vi "Dashboard Main.vi"() -> ()   [LabVIEW 2013]
uses:
  <vilib>/event_ctls.llb/eventvkey.ctl
  <vilib>/Utility/config.llb/Read Key (String).vi
  <vilib>/Utility/config.llb/Read Key (I32).vi
  <vilib>/Utility/config.llb/Write Key (String).vi
  <vilib>/Utility/config.llb/Write Key (I32).vi
  <vilib>/Utility/config.llb/NI_LVConfig.lvlib
panel:
  in  "Switches":bool
  out "Battery Value":dbl(slide) scale=0.0..14.0 scale format="%#_2e"
  out "Battery":sgl(graph)
  in  "Camera Settings":T1={"Frate Rate"=30, "Compression"=30, "Size"=1} {"Frate Rate" scale=1.0..30.0; "Size" items=["640x480", "320x240", "160x120"]}
  out "Mode":T2(ring)=enum."Auto Disabled"
  out "Camera IP":string
  out "JS1 Z":dbl(slide) scale=-1.0..1.0 scale format="%#_2e"
  out "JS2 Z":dbl(slide) scale=-1.0..1.0 scale format="%#_2e"
  out "Joystick 1":cluster{"X":dbl, "Y":dbl}[](graph)
  out "Joystick 2":cluster{"X":dbl, "Y":dbl}[](graph)
  out "JS Buttons 1":T3
  out "JS Buttons 2":T3
  out "MotorSlide4":dbl(slide) scale=-1.0..1.0 scale format="%#_2e"
  out "MotorSlide3":dbl(slide) scale=-1.0..1.0 scale format="%#_2e"
  out "MotorSlide2":dbl(slide) scale=-1.0..1.0 scale format="%#_2e"
  in  "MotorName3":string="Front Left"
  in  "MotorName4":string="Front Right"
  in  "MotorName1":string="Rear Left"
  in  "MotorName2":string="Rear Right"
  out "MotorChart4":dbl(graph)
  out "MotorChart3":dbl(graph)
  out "MotorChart2":dbl(graph)
  out "MotorSlide1":dbl(slide) scale=-1.0..1.0 scale format="%#_2e"
  out "MotorChart1":dbl(graph)
  out "Robot IP":string
  in  "Dashboard Tab":enum32{"Camera Image", "Test", "Checklist"}(tab)
  out "Right Claw 2":bool
  out "Left Claw":bool
  out "Right MAX":bool
  out "Left MAX":bool
  out "Shooter MIN":bool
  in  "Slider":dbl(slide) scale=0.0..100.0 scale format="%#_3g"
  in  "On/Off":bool caption="Solenoid"
  in  "Test Name":u16(ring) items=["Select the test to run...", "Example Test", "-------------------------------", "List of tests is built in robot code.", "Replace with your own automated tests."]
  in  "Test Tree":string(tree)
  in  "Motor":cluster{"Value":dbl, "Enable":bool} {"Value" scale=-1.0..1.0 scale format="%#_3g"}
  out "Progress":T4 {"Test Progress" scale=0.0..100.0}
  in  "Rev/Fwd":cluster{"Forward":bool, "Reverse":bool}
  in  "Ring":u16(ring) items=["Auto", "Fixed indoor", "Fixed outdoor 1", "Fixed outdoor 2", "Fixed fluorescent 1", "Fixed fluorescent 2", "Hold current"]
  in  "Listbox":i32(listbox)
  in  "Viewer":enum32{"Operation", "Variables"}(tab)
  out "Image Error Message":string="Timeout in Camera Communications"
  out "fps":dbl format="%#.1g"
  out "Mbps 2":bool
  in  "DB Camera Config":bool
  in  "Enable":bool
  out "Mbps":dbl format="%#.1g"
  out "Camera Image":T5(plugin-control)
  out "Tree":string(tree)
  # "Drive & Motors"
  # "Robot IP:"
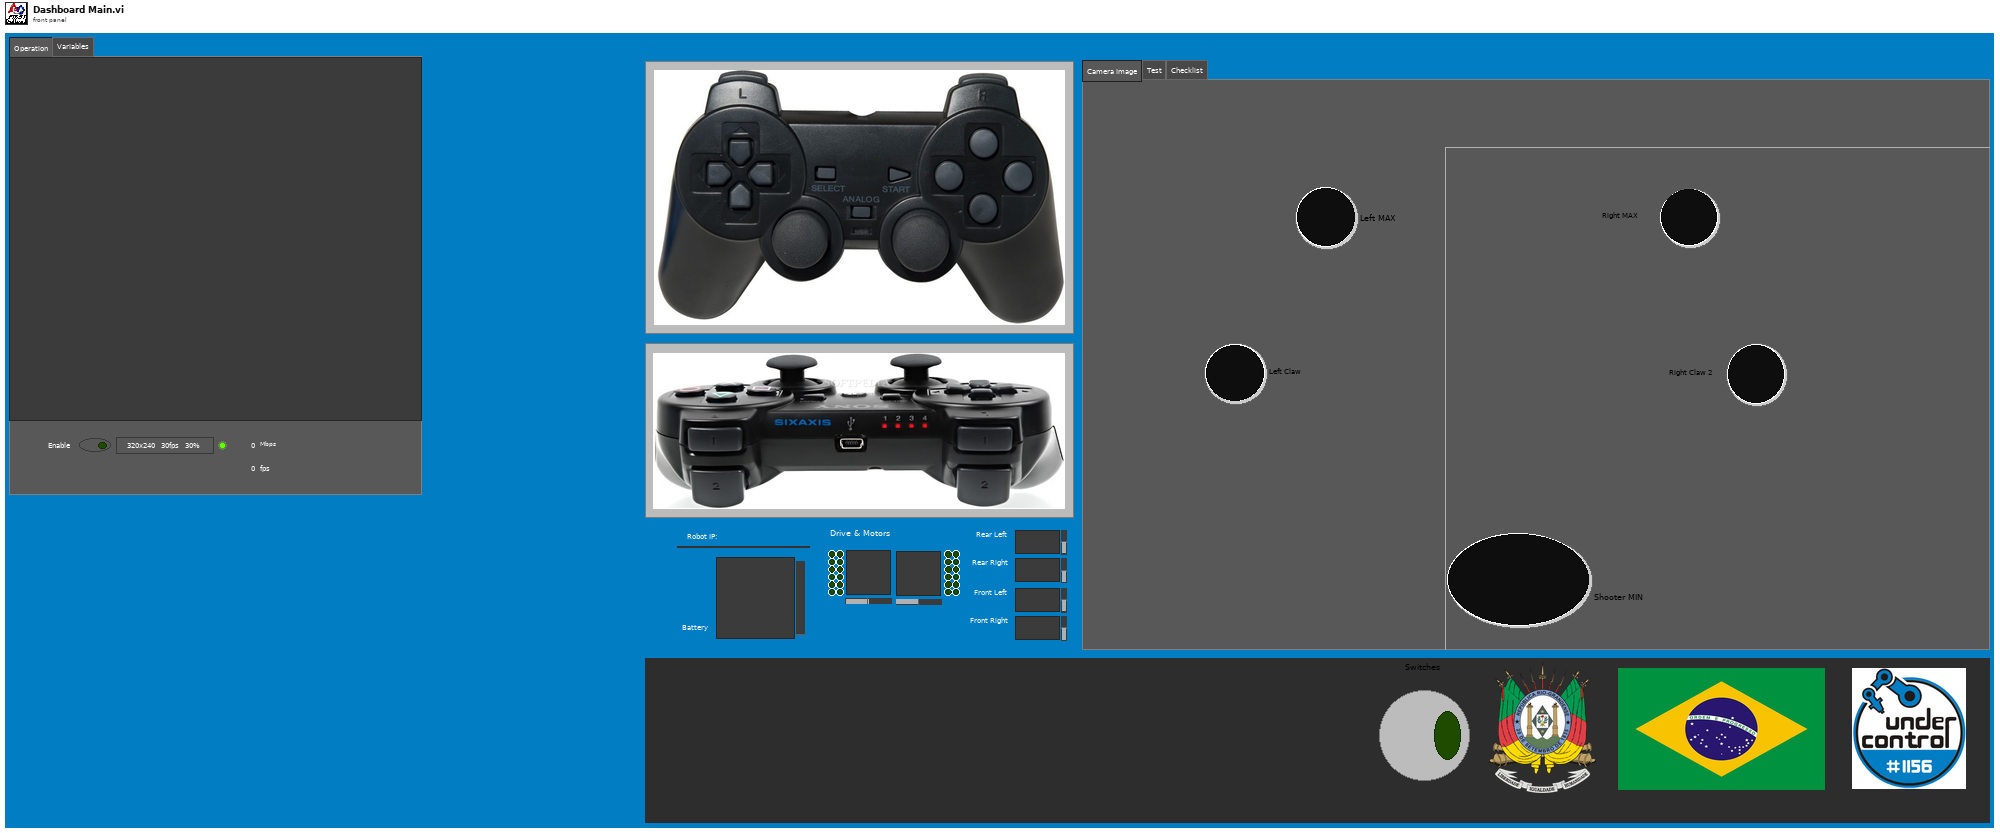
[diagram p1: front panel]
types:
  T1 = cluster{"Frate Rate":i32, "Compression":i32, "Size":u16}
  T2 = enum8{"Tele-Op Disabled", "Tele-Op Enabled", "Auto Disabled", "Auto Enabled", "Test Disabled", "Test Enabled", ""}
  T3 = cluster{bool, bool, bool, bool, bool, bool, bool, bool, bool, bool, bool, bool}
  T4 = cluster{"Test Progress":u8, "Test Progress Text":string}
  T5 = typedef "IMAQ Image.ctl" = refnum<image>
  T6 = typedef "Image Type" = u32
  T7 = typedef "LVRectTypeDef.ctl" = cluster{"Left":i16, "Top":i16, "Right":i16, "Bottom":i16}
  T8 = cluster{"Competition mode":bool, "Robot Link":bool, "Autonomous":bool, "Enabled":bool, "E-Stop":bool, "Simulated":bool, "TestMode":bool, "Docked Window":bool}
  T9 = cluster{"Boolean Array[0]":bool, "Boolean Array[1]":bool, "Boolean Array[2]":bool, "Boolean Array[3]":bool, "Boolean Array[4]":bool, "Boolean Array[5]":bool, "Boolean Array[6]":bool, "Boolean Array[7]":bool, "Boolean Array[8]":bool, "Boolean Array[9]":bool, "Boolean Array[10]":bool, "Boolean Array[11]":bool}
  T10 = typedef "NI_LVConfig.lvlib/Config Data RefNum.ctl" = refnum<k1>
  T11 = typedef "eventvkey.ctl" = enum16{"ASCII", "Enter", "Return", "Shift", "Ctrl", "Alt", "Cmd", "Opt", "Caps", "NumLock", "Clear", "Break", "Up", "Down", "Left", "Right", "Insert", "Delete", "Home", "End", "PageUp", "PageDown", "Escape", "Help", "Pause", "ScrollLock", "F1", "F2", "F3", "F4", "F5", "F6", "F7", "F8", "F9", "F10", "F11", "F12", "F13", "F14", "F15", "F16", "F17", "F18", "F19", "F20", "F21", "F22", "F23", "F24", "Play", "VolumeUp", "VolumeDown", "Mute", "Two Byte Char"}
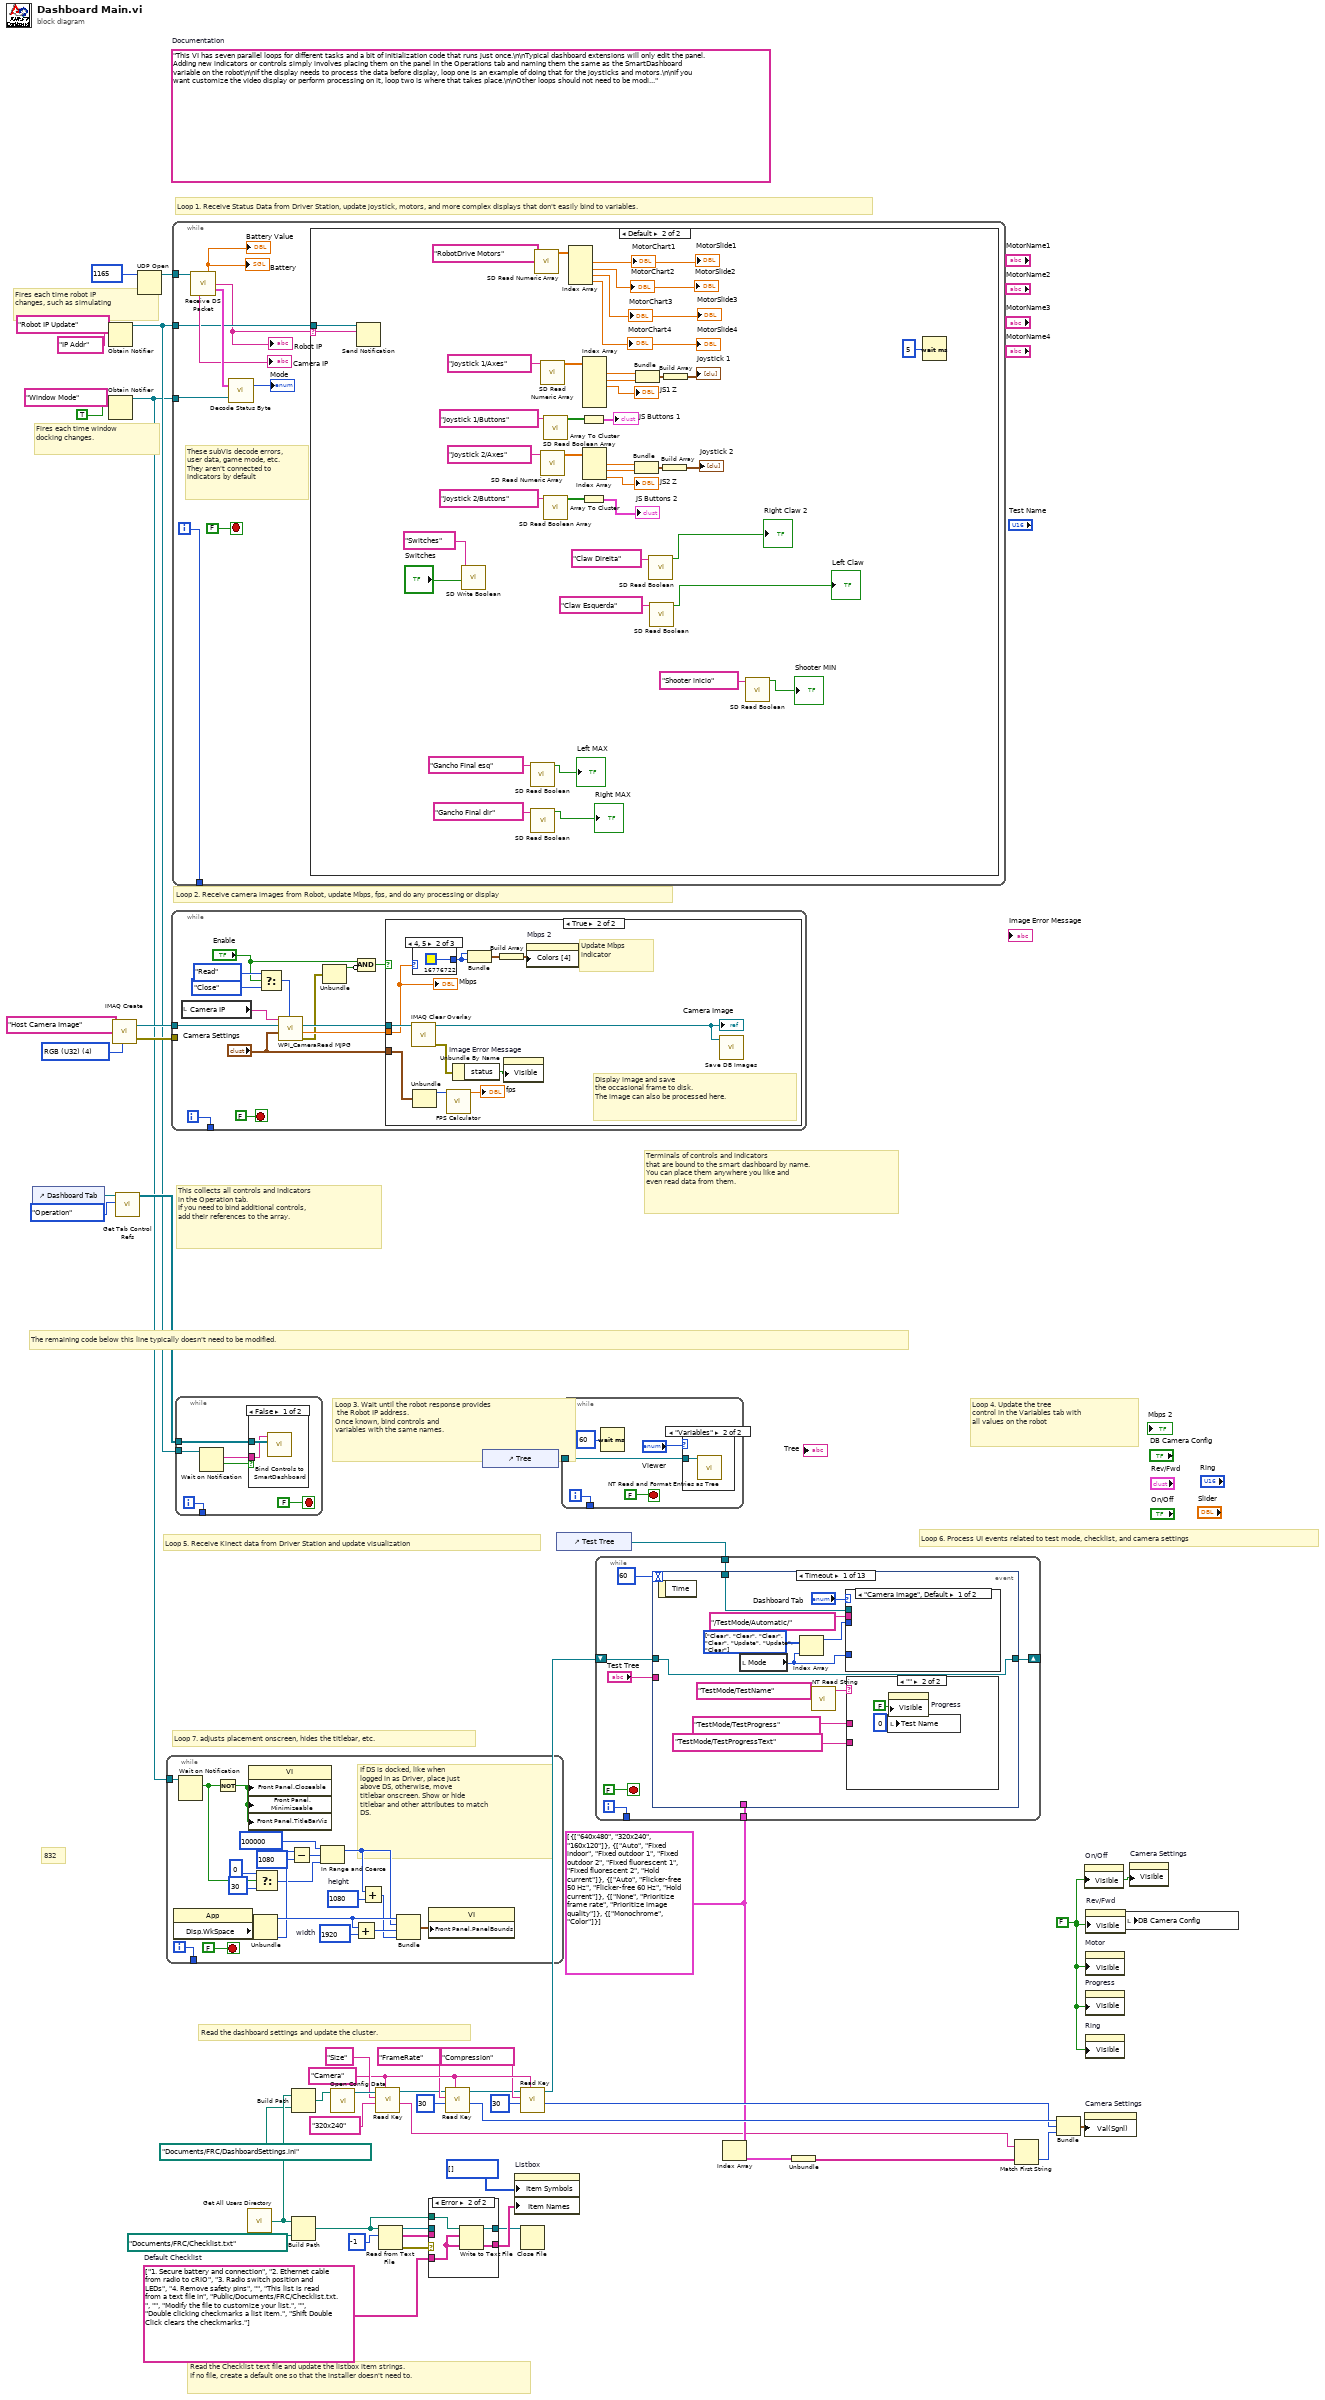
[diagram p0: block diagram]
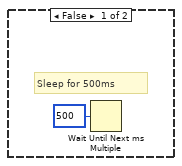
[diagram p3: hidden frame]
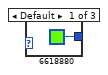
[diagram p4: hidden frame]
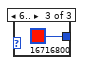
[diagram p5: hidden frame]
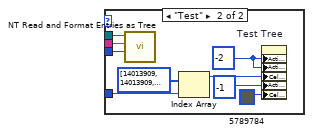
[diagram p7: hidden frame]
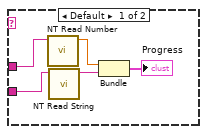
[diagram p8: hidden frame]
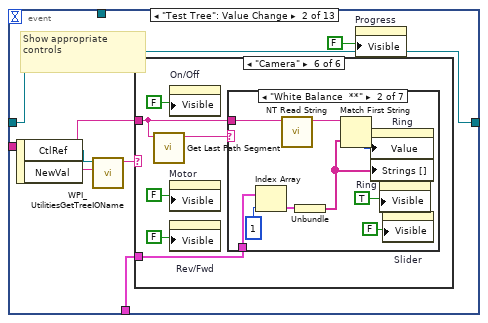
[diagram p9: hidden frame]
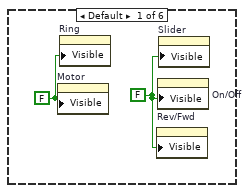
[diagram p10: hidden frame]
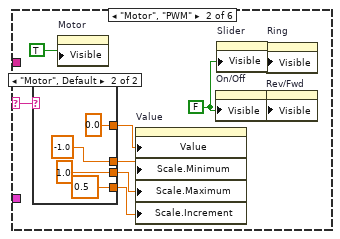
[diagram p11: hidden frame]
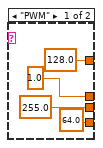
[diagram p12: hidden frame]
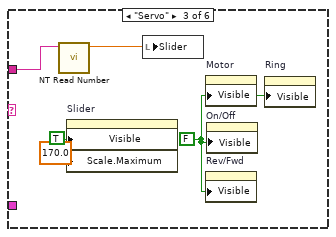
[diagram p13: hidden frame]
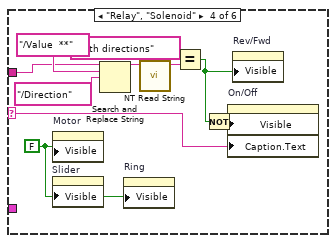
[diagram p14: hidden frame]
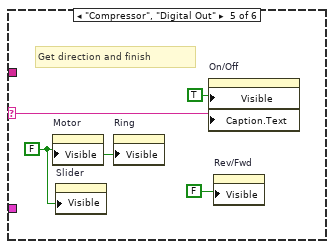
[diagram p15: hidden frame]
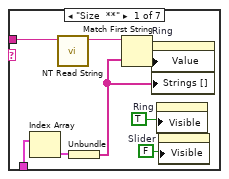
[diagram p16: hidden frame]
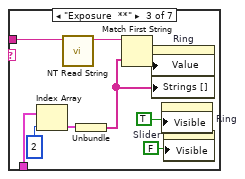
[diagram p17: hidden frame]
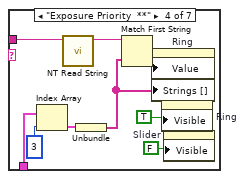
[diagram p18: hidden frame]
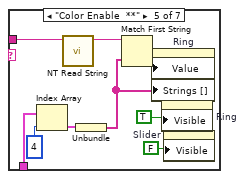
[diagram p19: hidden frame]
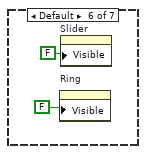
[diagram p20: hidden frame]
diagram:
  w21 = "Camera"
  w13 = cluster{string[]}[] [{["640x480", "320x240", "160x120"]}, {["Auto", "Fixed indoor", "Fixed outdoor 1", "Fixed outdoor 2", "Fixed fluorescent 1", "Fixed fluorescent 2", "Hold current"]}, {["Auto", "Flicker-free 50 Hz", "Flicker-free 60 Hz", "Hold current"]}, {["None", "Prioritize frame rate", "Prioritize image quality"]}, {["Monochrome", "Color"]}]
  w29 = string[] ["1. Secure battery and connection", "2. Ethernet cable from radio to cRIO", "3. Radio switch position and LEDs", "4. Remove safety pins", "", "This list is read from a text file in", "Public/Documents/FRC/Checklist.txt.", "", "Modify the file to customize your list.", "", "Double clicking checkmarks a list item.", "Shift Double Click clears the checkmarks."]  # Default Checklist
  w27 = FALSE ("Visible")
  (unwired) "This VI has seven parallel loops for different tasks and a bit of initialization code that runs just once.\n\nTypical dashboard extensions will only edit the panel. Adding new indicators or controls simply involves placing them on the panel in the Operations tab and naming them the same as the SmartDashboard variable on the robot\n\nIf the display needs to process the data before display, loop one is an example of doing that for the joysticks and motors.\n\nIf you want customize the video display or perform processing on it, loop two is where that takes place.\n\nOther loops should not need to be modified. They are pretty standard, and document the task they perform."  # Documentation
  w48 = T6 4 items=["Grayscale (U8)", "Grayscale (I16)", "Grayscale (SGL)", "Complex (CSG)", "RGB (U32)", "HSL (U32)", "RGB (U64)"] ("Image Type")
  # "832"
  # "Fires each time robot IP\nchanges, such as simulating"
  # "Fires each time window\ndocking changes."
  # "Read the Checklist text file and update the listbox item strings.\nIf no file, create a default one so that the installer doesn't need to."
  # "This collects all controls and indicators\nin the Operation tab.\nIf you need to bind additional controls,\nadd their references to the array."
  # "The remaining code below this line typically doesn't need to be modified."
  # "Loop 6. Process UI events related to test mode, checklist, and camera settings"
  # "Read the dashboard settings and update the cluster."
  # "Terminals of controls and indicators\nthat are bound to the smart dashboard by name.\nYou can place them anywhere you like and\neven read data from them."
  # "Loop 4. Update the tree\ncontrol in the Variables tab with\nall values on the robot"
  # "Loop 3. Wait until the robot response provides\n the Robot IP address.\nOnce known, bind controls and\nvariables with the same names."
  # "Loop 5. Receive Kinect data from Driver Station and update visualization"
  # "Loop 7. adjusts placement onscreen, hides the titlebar, etc."
  # "Loop 1. Receive Status Data from Driver Station, update joystick, motors, and more complex displays that don't easily bind to variables."
  # "Loop 2. Receive camera images from Robot, update Mbps, fps, and do any processing or display"
  n1 = control-ref of="Dashboard Tab"() -> (w43:refnum<vi>)
  n2 = Obtain Notifier(name (unnamed)="Robot IP Update", notification data type="IP Addr" ("name (unnamed)")) -> (notifier out=w40:refnum<notifier>)  [unwired: 2 in, 2 out]
  n3 = Obtain Notifier(name (unnamed)="Window Mode", notification data type=TRUE) -> (notifier out=w33:refnum<notifier>)  [unwired: 2 in, 2 out]
  n4 = call "IMAQ Create"("Image Name"="Host Camera Image", "Image Type"=w48) -> ("New Image"=w46:T5, "error out"=w45:errorcluster)  [unwired: 2 in, 1 out]
  n5 = call <vilib>:"Get Tab Control Refs.vi"("Page Index"=enum32{"Operation", "Test"}."Operation" ("Dashboard Tab"), "TabControl in"=w43) -> ("ControlsOnPage"=w44:refnum<vi>[])  [unwired: 9 in]
  n6 = UDP Open(11:u16 1165 ("port")) -> (port=w49:refnum<k16>)  [unwired: 2 in, 4 out]
  n7 = while {
    tunnel: w33 -> [w69]
    tunnel: [w67] -> _
    i -> [w67]
    stop <- FALSE stop-if-true
    w59 = 1920  # width
    w62 = 1080  # height
    # "If DS is docked, like when\nlogged in as Driver, place just\nabove DS, otherwise, move\ntitlebar onscreen. Show or hide\ntitlebar and other attributes to match\nDS."
    n8 = property class="App"() -> ("Disp.WkSpace"=w65:T7)  [unwired: 2 in, 2 out]
    n9 = Wait on Notification(notifier=w69) -> (notification=w54:bool)  [unwired: 3 in, 3 out]
    n10 = Not(x=w54) -> (.not. x?=w68:bool)
    n11 = property class="VI"("Front Panel.Closeable"=w68, "Front Panel.Minimizeable"=w68, "Front Panel.TitleBarVis"=w68) -> ()  [unwired: 2 in, 2 out]
    n12 = Unbundle(w65) -> ("Left"=w63:i16, "Bottom"=w60:i16)  [unwired: 2 out]
    n13 = Select(t=0, s=w54, f=30) -> (s? t:f=w53:i32)
    n14 = Subtract(x=w60, y=1080) -> (x-y=w57:i32)
    n15 = In Range and Coerce(upper limit=100000, x=w57, lower limit=w53) -> (coerced(x)=w51:i32)  [unwired: 1 out]
    n16 = Add(x=w63, y=w59) -> (x+y=w64:i32)
    n17 = Add(x=w51, y=w62) -> (x+y=w61:i32)
    n18 = Bundle("Left"=w63, w51, w64, w61) -> (w66:cluster{"Left":i16, i32, i32, i32})  [unwired: 1 out]
    n19 = property class="VI"("Front Panel.PanelBounds"=w66) -> ()  [unwired: 2 in, 2 out]
  }
  n20 = while {
    tunnel: w46 -> [w80]
    tunnel: w45 -> [_]
    tunnel: [w83] -> _
    i -> [w83]
    stop <- FALSE stop-if-true
    n21 = local read "Camera IP"() -> (w82:string)
    n22 = Select(t=enum16{"Read", "Reopen", "Close"}."Read" ("Operation"), s="Enable", f=enum16{"Read", "Reopen", "Close"}."Close" ("Operation")) -> (s? t:f=w75:enum16{"Read", "Reopen", "Close"})
    n23 = call <vilib>:"WPI_CameraRead MJPG.vi"("Operation"=w75, "Camera Settings"="Camera Settings", "Image"=w80, "address"=w82) -> ("error out"=w74:errorcluster, "Bandwidth (Mbps)"=w78:dbl, "Image Out"=w79:T5)  [unwired: 5 in]
    n24 = Unbundle(w74) -> ("status"=w72:bool)  [unwired: 2 out]
    n25 = Compound Arithmetic op=AND("Enable", invert w72) -> (w71:bool)
    n26 = case shown="True" w71 {
      tunnel: "Camera Settings" -> [_ w87]
      tunnel: w79 -> [_ w90]
      tunnel: w78 -> [_ w89]
      frame False {
        # "Sleep for 500ms"
        n27 = Wait Until Next ms Multiple(millisecond multiple=u32 500) -> ()  [unwired: 1 out]
      }
      frame True {
        # "Display image and save\nthe occasional frame to disk.\nThe image can also be processed here."
        # "Update Mbps\nindicator"
        n28 = call "IMAQ Clear Overlay"("Image"=w90) -> ("error out"=w95:errorcluster, "Image Out"=w94:T5)  [unwired: 2 in, 7 out]
        "Camera Image" <- w94
        n29 = case shown="4, 5" w89 {
          tunnel: [u32 6618880 ("Color Box") u32 16776722 ("Color Box") u32 16716800 ("Color Box")] -> w91
          frame Default {
          }
          frame 4, 5 {
          }
          frame 6.. {
          }
        }
        n30 = Unbundle(w87) -> ("Frate Rate"=w86:i32)  [unwired: 2 out]
        n31 = call "FPS Calculator.vi"("Average Count"=w86) -> ("fps"=→"fps":dbl)  [unwired: 10 in]
        n32 = Unbundle By Name(w95) -> ("status"=w96:bool)
        n33 = Bundle("Color Box"=w91, "Color Box"=w91) -> (w93:cluster{"Color Box":u32, "Color Box":u32})  [unwired: 1 out]
        n34 = Build Array(w93) -> (w92:cluster{"Color Box":u32, "Color Box":u32}[])
        n35 = property on="Image Error Message" class="Str"("Visible"=w96) -> ()  [unwired: 2 in, 2 out]
        n36 = property on="Mbps 2" class="Bool (strict)"("Colors [4]"=w92) -> ()  [unwired: 2 in, 2 out]
        n37 = call "Save DB Images.vi"("Image"=w94) -> ()  [unwired: 2 in, 1 out]
        "Mbps" <- w89
      }
    }
  }
  n38 = while {
    tunnel: w49 -> [w107]
    tunnel: w40 -> [w101]
    tunnel: w33 -> [w105]
    tunnel: [w102] -> _
    i -> [w102]
    stop <- FALSE stop-if-true
    # "These subVIs decode errors, user data, game mode, etc.\nThey aren't connected to indicators by default"
    n39 = call "Receive DS Packet.vi"("Recv Socket"=w107) -> ("Battery"=→"Battery" →"Battery Value":sgl, "Robot IP Address"=w100:string, "Status"=w108:T8, "Camera IP Address"=→"Camera IP":string)  [unwired: 1 in, 10 out]
    "Robot IP" <- w100
    n40 = call "Decode Status Byte.vi"("Window Mode Notifier"=w105, "Status"=w108) -> ("Mode"=→"Mode":T2)  [unwired: 1 out]
    n41 = case shown="Default" w100 {
      selector: w100 -> [_ w123]
      tunnel: w101 -> [_ w124]
      frame "0.0.0.0" {
        # "Robot not responding, don't poll the variables"
      }
      frame Default {
        n42 = Send Notification(notification=w123, notifier=w124) -> ()  [unwired: 1 in, 2 out]
        n43 = call <vilib>:"SD Write Boolean.vi"("Boolean"="Switches", "Name"="Switches") -> ()  [unwired: 8 in, 2 out]
        n44 = call <vilib>:"SD Read Boolean.vi"("Name"="Gancho Final esq") -> ("Boolean"=→"Left MAX":bool)  [unwired: 8 in, 2 out]
        n45 = call <vilib>:"SD Read Boolean.vi"("Name"="Gancho Final dir") -> ("Boolean"=→"Right MAX":bool)  [unwired: 8 in, 2 out]
        n46 = call <vilib>:"SD Read Numeric Array.vi"("Name"="RobotDrive Motors") -> ("Numeric Array"=w147:dbl[])  [unwired: 8 in, 2 out]
        n47 = call <vilib>:"SD Read Numeric Array.vi"("Name"="Joystick 1/Axes") -> ("Numeric Array"=w140:dbl[])  [unwired: 8 in, 2 out]
        n48 = call <vilib>:"SD Read Numeric Array.vi"("Name"="Joystick 2/Axes") -> ("Numeric Array"=w134:dbl[])  [unwired: 8 in, 2 out]
        n49 = call <vilib>:"SD Read Boolean Array.vi"("Name"="Joystick 1/Buttons") -> ("Boolean Array"=w142:bool[])  [unwired: 8 in, 2 out]
        n50 = call <vilib>:"SD Read Boolean Array.vi"("Name"="Joystick 2/Buttons") -> ("Boolean Array"=w133:bool[])  [unwired: 8 in, 2 out]
        n51 = Index Array(array=w147) -> (element #1=→"MotorChart1" →"MotorSlide1":dbl, element #2=→"MotorSlide2" →"MotorChart2":dbl, element #3=→"MotorChart3" →"MotorSlide3":dbl, element #4=→"MotorChart4" →"MotorSlide4":dbl)  [unwired: 4 in]
        n52 = Array To Cluster(array=w142) -> (cluster=→"JS Buttons 1":T9)
        n53 = Array To Cluster(array=w133) -> (cluster=→"JS Buttons 2":T9)
        n54 = Index Array(array=w140) -> (element #1=w137:dbl, element #2=w138:dbl, element #3=→"JS1 Z":dbl)  [unwired: 6 in, 3 out]
        n55 = Index Array(array=w134) -> (element #1=w129:dbl, element #2=w128:dbl, element #3=→"JS2 Z":dbl)  [unwired: 3 in]
        n56 = Bundle("Numeric"=w129, "Numeric"=w128) -> (w130:cluster{"Numeric":dbl, "Numeric":dbl})  [unwired: 1 in]
        n57 = Bundle("Numeric"=w137, "Numeric"=w138) -> (w136:cluster{"Numeric":dbl, "Numeric":dbl})  [unwired: 1 in]
        n58 = call <vilib>:"SD Read Boolean.vi"("Name"="Claw Direita") -> ("Boolean"=→"Right Claw 2":bool)  [unwired: 8 in, 2 out]
        n59 = call <vilib>:"SD Read Boolean.vi"("Name"="Claw Esquerda") -> ("Boolean"=→"Left Claw":bool)  [unwired: 8 in, 2 out]
        n60 = Build Array(w130) -> (→"Joystick 2":cluster{"Numeric":dbl, "Numeric":dbl}[])
        n61 = Build Array(w136) -> (→"Joystick 1":cluster{"Numeric":dbl, "Numeric":dbl}[])
        n62 = call <vilib>:"SD Read Boolean.vi"("Name"="Shooter inicio") -> ("Boolean"=→"Shooter MIN":bool)  [unwired: 8 in, 2 out]
        n63 = Wait (ms)(milliseconds to wait=u32 5) -> ()  [unwired: 1 out]
      }
    }
  }
  n64 = while {
    tunnel: w44 -> [w156]
    tunnel: w40 -> [w153]
    tunnel: [w151] -> _
    i -> [w151]
    stop <- FALSE stop-if-true
    n65 = Wait on Notification(notifier=w153) -> (notification=w152:string, timed out?=w154:bool)  [unwired: 3 in, 2 out]
    n66 = case shown="False" w154 {
      tunnel: w156 -> [w158 _]
      tunnel: w152 -> [w157 _]
      frame False {
        n67 = call <vilib>:"Bind Controls to SmartDashboard.vi"("Bound Control Refs"=w158, "Server IP Address"=w157) -> ()  [unwired: 10 in]
      }
      frame True {
      }
    }
  }
  n68 = call "Get All Users Directory.vi"() -> ("All User Path"=w26:path)
  n69 = Build Path(base path=w26, name or relative path=path "Documents/FRC/DashboardSettings.ini") -> (appended path=w25:path)
  n70 = Build Path(base path=w26, name or relative path=path "Documents/FRC/Checklist.txt") -> (appended path=w30:path)
  n71 = call <vilib>:"Open Config Data.vi"("configuration file path"=w25) -> ("refnum"=w24:T10)  [unwired: 8 in, 2 out]
  n72 = call-poly <vilib>:"Read Key.vi"("section"=w21, "default value"="320x240", "key"="Size", "refnum"=w24) -> ("value"=w11:string, "refnum out"=w6:T10)  [unwired: 2 in, 4 out]
  n73 = Read from Text File(file (use dialog)=w30, count=-1 ("timeout ms (25000)")) -> (refnum out=w8:refnum<file>, text=w31:string[], error out=w32:errorcluster)  [unwired: 2 in, 1 out]
  n74 = case shown="Error" w32 {
    tunnel: w31 -> [w160 _]
    tunnel: [w160 w162] -> w28
    tunnel: w29 -> [_ w162]
    tunnel: w30 -> [_ w163]
    tunnel: [w159 w161] -> w7
    tunnel: w8 -> [w159 _]
    frame No Error {
    }
    frame Error {
      n75 = Write to Text File(file (use dialog)=w163, text=w162) -> (refnum out=w161:refnum<file>)  [unwired: 2 in, 2 out]
    }
  }
  n76 = call-poly <vilib>:"Read Key.vi"("section"=w21, "default value"=30, "key"="FrameRate", "refnum"=w6) -> ("value"=w16:i32, "refnum out"=w5:T10)  [unwired: 1 in, 5 out]
  n77 = control-ref of="Tree"() -> (w2:refnum<vi>)
  n78 = property on="Listbox" class="LstBox (strict)"("Item Symbols"=i32[] [], "Item Names"=w28) -> ()  [unwired: 2 in, 2 out]
  n79 = Close File(refnum=w7) -> ()  [unwired: 1 in, 2 out]
  n80 = call-poly <vilib>:"Read Key.vi"("section"=w21, "default value"=30, "key"="Compression", "refnum"=w5) -> ("value"=w15:i32, "refnum out"=w3:T10)  [unwired: 1 in, 5 out]
  n81 = control-ref of="Test Tree"() -> (w1:refnum<vi>)
  n82 = while {
    tunnel: [w165] -> _
    tunnel: w2 -> [w164]
    i -> [w165]
    stop <- FALSE stop-if-true
    n83 = Wait (ms)(milliseconds to wait=u32 60) -> ()  [unwired: 1 out]
    n84 = case shown="\"Variables\"" "Viewer" {
      tunnel: w164 -> [_ w169]
      frame Default {
      }
      frame "Variables" {
        n85 = call <vilib>:"NT Read and Format Entries as Tree.vi"("Tree Refnum"=w169) -> ()  [unwired: 9 in, 2 out]
      }
    }
  }
  n86 = while {
    tunnel: w13 -> [w174]
    shift-right: [w173] -> _
    shift-left: w3 -> [w172]
    tunnel: [w171] -> _
    tunnel: w1 -> [w170]
    i -> [w171]
    stop <- FALSE stop-if-true
    n87 = event shown="[0] Timeout" {
      selector: _ -> [_ _ _ _ _ _ _ _ _ _ _ _ _]
      dyn-events: _ -> [_ _ _ _ _ _ _ _ _ _ _ _ _]
      timeout: u32 60 ("milliseconds to wait") -> [_ _ _ _ _ _ _ _ _ _ _ _ _]
      tunnel: w170 -> [w184 _ _ _ _ _ _ _ _ _ _ _ _]
      tunnel: "Test Tree" -> [_ _ _ _ _ _ _ _ w378 w386 w388 w392 w400]
      tunnel: w174 -> [_ w206 _ _ _ _ w342 w372 _ _ _ _ _]
      tunnel: [w178 w205 _ w308 w316 w328 w341 w365 w377 w384 w387 w391 w399] -> w173
      tunnel: w172 -> [w178 w205 _ w308 w316 w328 w340 w365 w377 w384 w387 w391 w399]
      event Timeout {
        w183 = enum16{"Update", "Clear"}[] [enum."Clear", enum."Clear", enum."Clear", enum."Clear", enum."Update", enum."Update", enum."Clear"] items=["Update", "Clear"]
        n88 = event-data() -> ()  [unwired: 1 in, 1 out]
        n89 = local read "Mode"() -> (w181:T2)
        n90 = Index Array(array=w183, index=w181) -> (element=w182:enum16{"Update", "Clear"})
        n91 = call <vilib>:"NT Read String.vi"("Name"="TestMode/TestName") -> ("String"=w187:string)  [unwired: 9 in, 1 out]
        n92 = case shown="\"Camera Image\", Default" "Dashboard Tab" {
          tunnel: w184 -> [_ w197]
          tunnel: "/TestMode/Automatic/" ("Name Pattern") -> [_ w196]
          tunnel: w182 -> [_ w195]
          tunnel: w181 -> [_ w193]
          frame "Camera Image", Default {
          }
          frame "Test" {
            w192 = -2 ("Active Item:Row Number")
            n93 = call <vilib>:"NT Read and Format Entries as Tree.vi"("Operation"=w195, "Name Pattern"=w196, "Tree Refnum"=w197) -> ()  [unwired: 7 in, 2 out]
            n94 = Index Array(array=u32[] [14013909, 14013909, 14013909, 14013909, 14013909, 16777215, 14013909], index=w193) -> (element=w191:u32)
            n95 = property on="Test Tree" class="Tree (strict)"("Active Item Row Number"=w192, "ActiveColNum"=w192, "CellBG"=w191, "Active Item Row Number"=-1 ("Active Item:Row Number"), "CellBG"=u32 5789784 ("Color Box")) -> ()  [unwired: 2 in, 2 out]
          }
        }
        n96 = case shown="\"\"" w187 {
          tunnel: "TestMode/TestProgress" ("Name") -> [w199 _]
          tunnel: "TestMode/TestProgressText" ("Name") -> [w198 _]
          frame Default {
            n97 = call <vilib>:"NT Read Number.vi"("Name"=w199) -> ("Numeric"=w200:dbl)  [unwired: 9 in, 1 out]
            n98 = call <vilib>:"NT Read String.vi"("Name"=w198) -> ("String"=w201:string)  [unwired: 9 in, 1 out]
            n99 = Bundle("Numeric"=w200, "String"=w201) -> (→"Progress":cluster{"Numeric":dbl, "String":string})  [unwired: 1 in]
          }
          frame "" {
            n100 = local write "Test Name"(u16 0) -> ()
            n101 = property on="Progress" class="Clust (strict)"("Visible"=FALSE) -> ()  [unwired: 2 in, 2 out]
          }
        }
      }
      event "Test Tree": Value Change {
        # "Show appropriate\ncontrols"
        n102 = event-data() -> ("CtlRef"=w209:refnum<vi>, "NewVal"=w207:string)  [unwired: 1 in]
        n103 = call <vilib>:"WPI_UtilitiesGetTreeIOName.vi"("NewVal"=w207, "TreeControl in"=w209) -> ("I/O Name"=w210:string)  [unwired: 9 in]
        n104 = case shown="\"Camera\"" w210 {
          selector: w210 -> [_ w217 _ w235 w244 _]
          tunnel: w207 -> [_ _ w232 w234 _ w251]
          tunnel: w206 -> [_ _ _ _ _ w250]
          frame Default {
            w212 = FALSE ("Visible")
            w211 = FALSE ("Visible")
            n105 = property on="Motor" class="Clust (strict)"("Visible"=w211) -> ()  [unwired: 2 in, 2 out]
            n106 = property on="Ring" class="Ring (strict)"("Visible"=w211) -> ()  [unwired: 2 in, 2 out]
            n107 = property on="Rev/Fwd" class="Clust (strict)"("Visible"=w212) -> ()  [unwired: 2 in, 2 out]
            n108 = property on="On/Off" class="Bool (strict)"("Visible"=w212) -> ()  [unwired: 2 in, 2 out]
            n109 = property on="Slider" class="Slide (strict)"("Visible"=w212) -> ()  [unwired: 2 in, 2 out]
          }
          frame "Motor", "PWM" {
            w218 = FALSE ("Visible")
            n110 = case shown="\"Motor\", Default" w217 {
              tunnel: [1.0 ("Value") -1.0 ("Value")] -> w216
              tunnel: [255.0 ("Value") 1.0 ("Value")] -> w215
              tunnel: [128.0 ("Value") 0.0 ("Value")] -> w214
              tunnel: [64.0 ("Value") 0.5 ("Value")] -> w213
              frame "PWM" {
              }
              frame "Motor", Default {
              }
            }
            n111 = property on="Motor" class="Clust (strict)"("Visible"=TRUE) -> ()  [unwired: 2 in, 2 out]
            n112 = property on="Value" class="Slide (strict)"("Value"=w214, "Scale.Minimum"=w216, "Scale.Maximum"=w215, "Scale.Increment"=w213) -> ()  [unwired: 2 in, 2 out]
            n113 = property on="On/Off" class="Bool (strict)"("Visible"=w218) -> ()  [unwired: 2 in, 2 out]
            n114 = property on="Slider" class="Slide (strict)"("Visible"=w218) -> ()  [unwired: 2 in, 2 out]
            n115 = property on="Ring" class="Ring (strict)"("Visible"=w218) -> ()  [unwired: 2 in, 2 out]
            n116 = property on="Rev/Fwd" class="Clust (strict)"("Visible"=w218) -> ()  [unwired: 2 in, 2 out]
          }
          frame "Servo" {
            w230 = FALSE ("Visible")
            n117 = call <vilib>:"NT Read Number.vi"("Name"=w232) -> ("Numeric"=w231:dbl)  [unwired: 9 in, 1 out]
            n118 = property on="Slider" class="Slide (strict)"("Visible"=TRUE, "Scale.Maximum"=170.0 ("Scale.Range:Maximum")) -> ()  [unwired: 2 in, 2 out]
            n119 = local write "Slider"(w231) -> ()
            n120 = property on="Motor" class="Clust (strict)"("Visible"=w230) -> ()  [unwired: 2 in, 2 out]
            n121 = property on="Rev/Fwd" class="Clust (strict)"("Visible"=w230) -> ()  [unwired: 2 in, 2 out]
            n122 = property on="On/Off" class="Bool (strict)"("Visible"=w230) -> ()  [unwired: 2 in, 2 out]
            n123 = property on="Ring" class="Ring (strict)"("Visible"=w230) -> ()  [unwired: 2 in, 2 out]
          }
          frame "Relay", "Solenoid" {
            w233 = FALSE ("Visible")
            n124 = property on="Motor" class="Clust (strict)"("Visible"=w233) -> ()  [unwired: 2 in, 2 out]
            n125 = property on="Slider" class="Slide (strict)"("Visible"=w233) -> ()  [unwired: 2 in, 2 out]
            n126 = Search and Replace String(input string=w234, search string="/Value  **", replace string="/Direction") -> (result string=w240:string)  [unwired: 5 in, 3 out]
            n127 = property on="Ring" class="Ring (strict)"("Visible"=w233) -> ()  [unwired: 2 in, 2 out]
            n128 = call <vilib>:"NT Read String.vi"("Name"=w240) -> ("String"=w238:string)  [unwired: 9 in, 1 out]
            n129 = Equal?(x="Both directions", y=w238) -> (x = y?=w236:bool)
            n130 = Not(x=w236) -> (.not. x?=w237:bool)
            n131 = property on="On/Off" class="Bool (strict)"("Visible"=w237, "Caption.Text"=w235) -> ()  [unwired: 2 in, 2 out]
            n132 = property on="Rev/Fwd" class="Clust (strict)"("Visible"=w236) -> ()  [unwired: 2 in, 2 out]
          }
          frame "Compressor", "Digital Out" {
            w243 = FALSE ("Visible")
            # "Get direction and finish"
            n133 = property on="Motor" class="Clust (strict)"("Visible"=w243) -> ()  [unwired: 2 in, 2 out]
            n134 = property on="Slider" class="Slide (strict)"("Visible"=w243) -> ()  [unwired: 2 in, 2 out]
            n135 = property on="Ring" class="Ring (strict)"("Visible"=w243) -> ()  [unwired: 2 in, 2 out]
            n136 = property on="On/Off" class="Bool (strict)"("Visible"=TRUE, "Caption.Text"=w244) -> ()  [unwired: 2 in, 2 out]
            n137 = property on="Rev/Fwd" class="Clust (strict)"("Visible"=FALSE) -> ()  [unwired: 2 in, 2 out]
          }
          frame "Camera" {
            n138 = call <vilib>:"Get Last Path Segment.vi"("String in"=w251) -> ("String out"=w252:string)  [unwired: 10 in]
            n139 = property on="On/Off" class="Bool (strict)"("Visible"=FALSE) -> ()  [unwired: 2 in, 2 out]
            n140 = property on="Motor" class="Clust (strict)"("Visible"=FALSE) -> ()  [unwired: 2 in, 2 out]
            n141 = property on="Rev/Fwd" class="Clust (strict)"("Visible"=FALSE) -> ()  [unwired: 2 in, 2 out]
            n142 = case shown="\"White Balance  **\"" w252 {
              tunnel: w251 -> [w258 w267 w276 w285 w294 _ w300]
              tunnel: w250 -> [w256 w264 w273 w282 w291 _ _]
              frame "Size  **" {
                n143 = Index Array(array=w256) -> (element=w255:cluster{string[]})  [unwired: 1 in]
                n144 = call <vilib>:"NT Read String.vi"("Name"=w258) -> ("String"=w257:string)  [unwired: 9 in, 1 out]
                n145 = Unbundle(w255) -> (w253:string[])
                n146 = Match First String(2:w253, 3:w257) -> (0:w254:i32)  [unwired: 1 out]
                n147 = property on="Ring" class="Ring (strict)"("Value"=w254, "Strings []"=w253) -> ()  [unwired: 2 in, 2 out]
                n148 = property on="Ring" class="Ring (strict)"("Visible"=TRUE) -> ()  [unwired: 2 in, 2 out]
                n149 = property on="Slider" class="Slide (strict)"("Visible"=FALSE) -> ()  [unwired: 2 in, 2 out]
              }
              frame "White Balance  **" {
                n150 = Index Array(array=w264, index=1) -> (element=w265:cluster{string[]})
                n151 = call <vilib>:"NT Read String.vi"("Name"=w267) -> ("String"=w266:string)  [unwired: 9 in, 1 out]
                n152 = Unbundle(w265) -> (w262:string[])
                n153 = Match First String(2:w262, 3:w266) -> (0:w261:i32)  [unwired: 1 out]
                n154 = property on="Ring" class="Ring (strict)"("Value"=w261, "Strings []"=w262) -> ()  [unwired: 2 in, 2 out]
                n155 = property on="Ring" class="Ring (strict)"("Visible"=TRUE) -> ()  [unwired: 2 in, 2 out]
                n156 = property on="Slider" class="Slide (strict)"("Visible"=FALSE) -> ()  [unwired: 2 in, 2 out]
              }
              frame "Exposure  **" {
                n157 = Index Array(array=w273, index=2) -> (element=w274:cluster{string[]})
                n158 = call <vilib>:"NT Read String.vi"("Name"=w276) -> ("String"=w275:string)  [unwired: 9 in, 1 out]
                n159 = Unbundle(w274) -> (w270:string[])
                n160 = Match First String(2:w270, 3:w275) -> (0:w271:i32)  [unwired: 1 out]
                n161 = property on="Ring" class="Ring (strict)"("Value"=w271, "Strings []"=w270) -> ()  [unwired: 2 in, 2 out]
                n162 = property on="Ring" class="Ring (strict)"("Visible"=TRUE) -> ()  [unwired: 2 in, 2 out]
                n163 = property on="Slider" class="Slide (strict)"("Visible"=FALSE) -> ()  [unwired: 2 in, 2 out]
              }
              frame "Exposure Priority  **" {
                n164 = Index Array(array=w282, index=3) -> (element=w283:cluster{string[]})
                n165 = call <vilib>:"NT Read String.vi"("Name"=w285) -> ("String"=w284:string)  [unwired: 9 in, 1 out]
                n166 = Unbundle(w283) -> (w279:string[])
                n167 = Match First String(2:w279, 3:w284) -> (0:w280:i32)  [unwired: 1 out]
                n168 = property on="Ring" class="Ring (strict)"("Value"=w280, "Strings []"=w279) -> ()  [unwired: 2 in, 2 out]
                n169 = property on="Ring" class="Ring (strict)"("Visible"=TRUE) -> ()  [unwired: 2 in, 2 out]
                n170 = property on="Slider" class="Slide (strict)"("Visible"=FALSE) -> ()  [unwired: 2 in, 2 out]
              }
              frame "Color Enable  **" {
                n171 = Index Array(array=w291, index=4) -> (element=w292:cluster{string[]})
                n172 = call <vilib>:"NT Read String.vi"("Name"=w294) -> ("String"=w293:string)  [unwired: 9 in, 1 out]
                n173 = Unbundle(w292) -> (w288:string[])
                n174 = Match First String(2:w288, 3:w293) -> (0:w289:i32)  [unwired: 1 out]
                n175 = property on="Ring" class="Ring (strict)"("Value"=w289, "Strings []"=w288) -> ()  [unwired: 2 in, 2 out]
                n176 = property on="Ring" class="Ring (strict)"("Visible"=TRUE) -> ()  [unwired: 2 in, 2 out]
                n177 = property on="Slider" class="Slide (strict)"("Visible"=FALSE) -> ()  [unwired: 2 in, 2 out]
              }
              frame Default {
                n178 = property on="Ring" class="Ring (strict)"("Visible"=FALSE) -> ()  [unwired: 2 in, 2 out]
                n179 = property on="Slider" class="Slide (strict)"("Visible"=FALSE) -> ()  [unwired: 2 in, 2 out]
              }
              frame "Brightness  **", "Color Level  **", "Compression  **", "FPS  **", "Sharpness  **" {
                n180 = call <vilib>:"NT Read Number.vi"("Name"=w300) -> ("Numeric"=w299:dbl)  [unwired: 9 in, 1 out]
                n181 = local write "Slider"(w299) -> ()
                n182 = property on="Slider" class="Slide (strict)"("Visible"=TRUE, "Scale.Maximum"=100.0 ("Scale.Range:Maximum")) -> ()  [unwired: 2 in, 2 out]
                n183 = property on="Ring" class="Ring (strict)"("Visible"=FALSE) -> ()  [unwired: 2 in, 2 out]
              }
            }
          }
        }
        n184 = property on="Progress" class="Clust (strict)"("Visible"=FALSE) -> ()  [unwired: 2 in, 2 out]
      }
      event "Test Name": Mouse Enter {
        # "Populate the ring with the list of tests"
        n185 = event-data() -> ()  [unwired: 1 in, 1 out]
        n186 = call <vilib>:"NT Read String Array.vi"("Name"="TestMode/TestList") -> ("String Array"=w307:string[])  [unwired: 9 in, 1 out]
        n187 = Build Array (concatenate)("Select the test to run...", w307) -> (w306:string[])
        n188 = property on="Test Name" class="Ring (strict)"("Strings []"=w306) -> ()  [unwired: 2 in, 2 out]
      }
      event "Test Name": Value Change {
        w309 = FALSE ("Visible")
        # "Tell the robot the test name to run"
        n189 = event-data() -> ("NewVal"=w313:u16)  [unwired: 1 in]
        n190 = property on="Test Name" class="Ring (strict)"() -> ("Strings []"=w314:string[])  [unwired: 2 in, 2 out]
        n191 = local write "Progress"(T4 {"Test Progress"=0, "Test Progress Text"=""} ("Progress")) -> ()
        n192 = Index Array(array=w314, index=w313) -> (element=w312:string)
        n193 = call <vilib>:"NT Write String.vi"("String"=w312, "Name"="TestMode/TestName") -> ()  [unwired: 9 in, 1 out]
        n194 = property on="Progress" class="Clust (strict)"("Visible"=TRUE) -> ()  [unwired: 2 in, 2 out]
        n195 = property on="Motor" class="Clust (strict)"("Visible"=w309) -> ()  [unwired: 2 in, 2 out]
        n196 = property on="Slider" class="Slide (strict)"("Visible"=w309) -> ()  [unwired: 2 in, 2 out]
        n197 = property on="On/Off" class="Bool (strict)"("Visible"=w309) -> ()  [unwired: 2 in, 2 out]
        n198 = property on="Rev/Fwd" class="Clust (strict)"("Visible"=w309) -> ()  [unwired: 2 in, 2 out]
        n199 = property on="Ring" class="Ring (strict)"("Visible"=w309) -> ()  [unwired: 2 in, 2 out]
      }
      event "Listbox": Double Click {
        n200 = event-data() -> ("PlatMods.Shift"=w317:bool, "Row"=w319:i32)  [unwired: 1 in]
        n201 = case shown="False" w317 {
          tunnel: w319 -> [w323 _]
          tunnel: 1 -> [w322 _]
          frame False {
            n202 = property on="Listbox" class="LstBox (strict)"() -> ("Item Symbols"=w321:i32[])  [unwired: 2 in, 2 out]
            n203 = Replace Array Subset(array=w321, new element=w322, index=w323) -> (w320:i32[])
            n204 = property on="Listbox" class="LstBox (strict)"("Item Symbols"=w320) -> ()  [unwired: 2 in, 2 out]
          }
          frame True {
            w324 = 0 ("Top Row")
            n205 = property on="Listbox" class="LstBox (strict)"() -> ("Number of Rows"=w326:u32)  [unwired: 2 in, 2 out]
            n206 = Initialize Array(0, w326) -> (w325:i32[])
            n207 = property on="Listbox" class="LstBox (strict)"("Top Row"=w324, "Value"=w324, "Item Symbols"=w325) -> ()  [unwired: 2 in, 2 out]
          }
        }
      }
      event "Listbox": Key Down {
        n208 = event-data() -> ("VKey"=w330:T11)  [unwired: 1 in]
        n209 = case shown="\"Left\", \"Right\"" w330 {
          selector: w330 -> [w335 _]
          tunnel: eventvkey."Left" ("VKey") -> [w333 _]
          frame "Left", "Right" {
            n210 = Equal?(x=w333, y=w335) -> (x = y?=w334:bool)
            n211 = Select(t=0, s=w334, f=1) -> (s? t:f=w336:i32)
            n212 = property on="Listbox" class="LstBox (strict)"() -> ("Item Symbols"=w339:i32[])  [unwired: 2 in, 2 out]
            n213 = Replace Array Subset(array=w339, new element=w336, index="Listbox") -> (w338:i32[])
            n214 = property on="Listbox" class="LstBox (strict)"("Item Symbols"=w338) -> ()  [unwired: 2 in, 2 out]
          }
          frame Default {
          }
        }
      }
      event "DB Camera Config": Value Change {
        n215 = event-data() -> ("NewVal"=w343:bool)  [unwired: 1 in]
        n216 = case shown="False" w343 {
          tunnel: w342 -> [w352 _]
          tunnel: [w345 w363] -> w341
          tunnel: w340 -> [w344 w363]
          frame False {
            w359 = "Camera"
            w362 = FALSE ("Visible")
            n217 = local read "Camera Settings"() -> (w351:T1)
            n218 = Index Array(array=w352) -> (element=w355:cluster{string[]})  [unwired: 1 in]
            n219 = Unbundle(w351) -> ("Frate Rate"=w350:i32, "Compression"=w349:i32, "Size"=w353:u16)
            n220 = Unbundle(w355) -> (w354:string[])
            n221 = Index Array(array=w354, index=w353) -> (element=w348:string)
            n222 = call-poly <vilib>:"Write Key.vi"("section"=w359, "value"=w348, "key"="Size", "refnum"=w344) -> ("refnum out"=w361:T10)  [unwired: 2 in, 5 out]
            n223 = call-poly <vilib>:"Write Key.vi"("section"=w359, "value"=w350, "key"="FrameRate", "refnum"=w361) -> ("refnum out"=w360:T10)  [unwired: 1 in, 6 out]
            n224 = local write "DB Camera Config"(w362) -> ()
            n225 = property on="Camera Settings" class="Clust (strict)"("Visible"=w362) -> ()  [unwired: 2 in, 2 out]
            n226 = call-poly <vilib>:"Write Key.vi"("section"=w359, "value"=w349, "key"="Compression", "refnum"=w360) -> ("refnum out"=w346:T10)  [unwired: 1 in, 6 out]
            n227 = call <vilib>:"Close Config Data.vi"("refnum"=w346) -> ("file path"=w347:path)  [unwired: 2 in, 8 out]
            n228 = call <vilib>:"Open Config Data.vi"("configuration file path"=w347) -> ("refnum"=w345:T10)  [unwired: 8 in, 2 out]
          }
          frame True {
            n229 = property on="Camera Settings" class="Clust (strict)"("Visible"=TRUE) -> ()  [unwired: 2 in, 2 out]
          }
        }
      }
      event "Camera Settings": Value Change {
        n230 = event-data() -> ("NewVal"=w376:T1)  [unwired: 1 in]
        n231 = Index Array(array=w372) -> (element=w371:cluster{string[]})  [unwired: 1 in]
        n232 = Unbundle(w376) -> ("Frate Rate"=w367:i32, "Compression"=w366:i32, "Size"=w369:u16)
        n233 = Unbundle(w371) -> (w370:string[])
        n234 = Index Array(array=w370, index=w369) -> (element=w368:string)
        n235 = Format Into String(format string="%s   %dfps   %d%%", w368, w367, w366) -> (resulting string=w373:string)  [unwired: 2 in, 1 out]
        n236 = Build Array(w373) -> (w374:string[])
        n237 = property on="DB Camera Config" class="Bool (strict)"("Strings [4]"=w374) -> ()  [unwired: 2 in, 2 out]
      }
      event "Motor.Enable": Value Change {
        n238 = event-data() -> ("NewVal"=w382:bool)  [unwired: 1 in]
        n239 = Unbundle("Motor") -> ("Value"=w381:dbl)  [unwired: 1 out]
        n240 = Select(t=w381, s=w382, f=0.0) -> (s? t:f=w379:dbl)
        n241 = call <vilib>:"NT Write Number.vi"("Numeric"=w379, "Name"=w378) -> ()  [unwired: 9 in, 1 out]
      }
      event "Slider": Value Change {
        n242 = event-data() -> ("NewVal"=w385:dbl)  [unwired: 1 in]
        n243 = call <vilib>:"NT Write Number.vi"("Numeric"=w385, "Name"=w386) -> ()  [unwired: 9 in, 1 out]
      }
      event "On/Off": Value Change {
        n244 = event-data() -> ("NewVal"=w390:bool)  [unwired: 1 in]
        n245 = Boolean To (0,1)(Boolean=w390) -> (0, 1=w389:i16)
        n246 = call <vilib>:"NT Write Number.vi"("Numeric"=w389, "Name"=w388) -> ()  [unwired: 9 in, 1 out]
      }
      event "Rev/Fwd": Value Change {
        n247 = event-data() -> ("NewVal.Forward"=w398:bool, "NewVal.Reverse"=w397:bool)  [unwired: 1 in]
        n248 = Boolean To (0,1)(Boolean=w398) -> (0, 1=w394:i16)
        n249 = Boolean To (0,1)(Boolean=w397) -> (0, 1=w396:i16)
        n250 = Negate(x=w396) -> (-x=w395:i16)
        n251 = Add(x=w394, y=w395) -> (x+y=w393:i16)
        n252 = call <vilib>:"NT Write Number.vi"("Numeric"=w393, "Name"=w392) -> ()  [unwired: 9 in, 1 out]
      }
      event "Ring": Value Change {
        n253 = event-data() -> ("NewVal"=w402:u16)  [unwired: 1 in]
        n254 = property on="Ring" class="Ring (strict)"() -> ("Strings []"=w403:string[])  [unwired: 2 in, 2 out]
        n255 = Index Array(array=w403, index=w402) -> (element=w401:string)
        n256 = call <vilib>:"NT Write String.vi"("String"=w401, "Name"=w400) -> ()  [unwired: 9 in, 1 out]
      }
    }
  }
  n257 = Index Array(array=w13) -> (element=w14:cluster{string[]})  [unwired: 1 in]
  n258 = Unbundle(w14) -> (w12:string[])
  n259 = Match First String(2:w12, 3:w11) -> (0:w10:i32)  [unwired: 1 out]
  n260 = Bundle("value"=w16, "value"=w15, "index"=w10) -> (w4:cluster{"value":i32, "value":i32, "index":i32})  [unwired: 1 out]
  n261 = property on="On/Off" class="Bool (strict)"("Visible"=w27) -> ()  [unwired: 2 in, 2 out]
  n262 = property on="Camera Settings" class="Clust (strict)"("Val(Sgnl)"=w4) -> ()  [unwired: 2 in, 2 out]
  n263 = property on="Motor" class="Clust (strict)"("Visible"=w27) -> ()  [unwired: 2 in, 2 out]
  n264 = property on="Progress" class="Clust (strict)"("Visible"=w27) -> ()  [unwired: 2 in, 2 out]
  n265 = property on="Ring" class="Ring (strict)"("Visible"=w27) -> ()  [unwired: 2 in, 2 out]
  n266 = property on="Rev/Fwd" class="Clust (strict)"("Visible"=w27) -> ()  [unwired: 2 in, 2 out]
  n267 = local write "DB Camera Config"(w27) -> ()
  n268 = property on="Camera Settings" class="Clust (strict)"("Visible"=w27) -> ()  [unwired: 2 in, 2 out]
